vi "Log Data to File.vi"(8 "error in (no error)":errorcluster, 9 "device_id":string="0", 10 "Data to log":waveform(dbl)[](array[waveform])=[{"t0"=timestamp(3726935017.7893386 s since 1904-01-01), "dt"=1.0, "Y"=[270.81512140186686], "attributes"=variant("NI_ChannelName"=variant(string "Ch 0"))}, {"t0"=timestamp(3726935017.7893386 s since 1904-01-01), "dt"=1.0, "Y"=[271.15098549836745], "attributes"=variant("NI_ChannelName"=variant(string "Ch 1"))}, {"t0"=timestamp(3726935017.7893386 s since 1904-01-01), "dt"=1.0, "Y"=[272.0245652598647], "attributes"=variant("NI_ChannelName"=variant(string "Ch 2"))}], 11 "TDMS File Reference":refnum<k34>) -> (0 "error out":errorcluster)   [LabVIEW 2019, in "Logger.lvlib"]
doc: "This VI uses the TDMS Write function to write data to a TDMS file.\n_____\nBased on DQMH Project Template 6.0.0.91."
uses:
  Logger.lvlib
  <vilib>/Utility/file.llb/Write Delimited Spreadsheet (DBL).vi
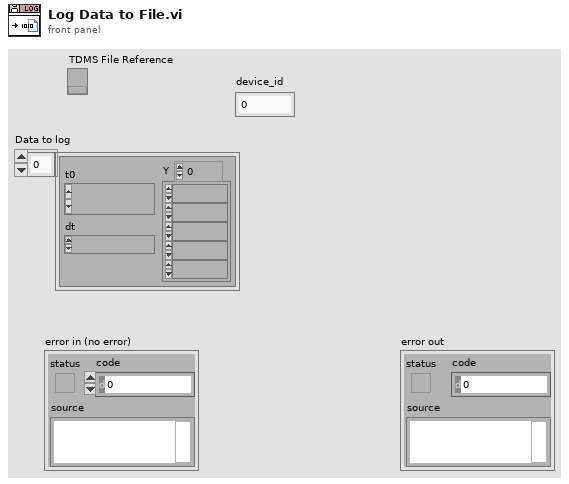
[diagram p1: front panel]
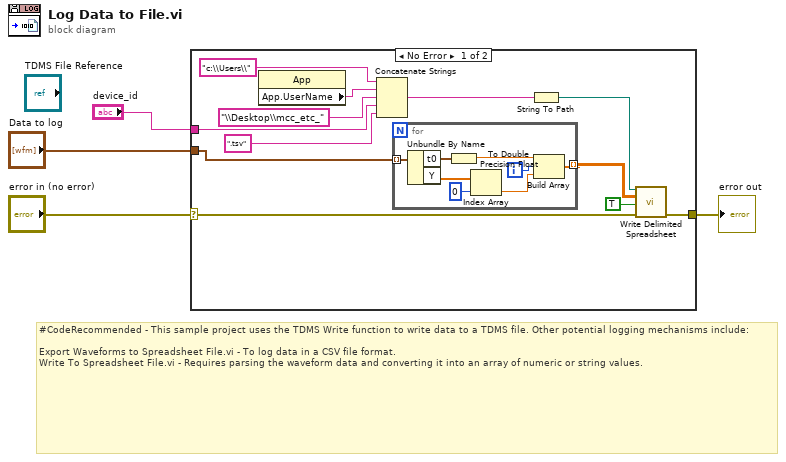
[diagram p0: block diagram]
diagram:
  # "#CodeRecommended - This sample project uses the TDMS Write function to write data to a TDMS file. Other potential logging mechanisms include:\n\nExport Waveforms to Spreadsheet File.vi - To log data in a CSV file format.\nWrite To Spreadsheet File.vi - Requires parsing the waveform data and converting it into an array of numeric or string values."
  n1 = case shown="No Error" "error in (no error)" {
    selector: "error in (no error)" -> [w9 w25]
    tunnel: "Data to log" -> [w8 _]
    tunnel: [w10 w25] -> w3
    tunnel: "device_id" -> [w6 _]
    frame No Error {
      n2 = property class="App"() -> ("App.UserName"=w15:string)  [unwired: 2 in, 2 out]
      n3 = Concatenate Strings("c:\\Users\\", w15, "\\Desktop\\mcc_etc_", w6, ".tsv") -> (w13:string)
      n4 = for {
        tunnel: w8 -> [w24] mode=indexing
        tunnel: [w23] -> w7 mode=indexing
        i -> [w20]
        n5 = Unbundle By Name(w24) -> ("t0"=w22:timestamp, "Y"=w19:dbl[])
        n6 = To Double Precision Float(number=w22) -> (double precision float=w21:dbl)
        n7 = Index Array(array=w19, index=0) -> (element=w17:dbl)
        n8 = Build Array(w21, w20, w17) -> (w23:dbl[])
      }
      n9 = String To Path(string=w13) -> (path=w11:path)
      n10 = call-poly <vilib>:"Write Delimited Spreadsheet.vi"("file path (dialog if empty)"=w11, "2D data"=w7, "append to file? (new file:F)"=TRUE, "error in (no error)"=w9) -> ("error out"=w10:errorcluster)  [unwired: 10 in, 1 out]
    }
    frame Error {
    }
  }
  "error out" <- w3
